vi "Load Default Configuration.vi"(8 "error in (no error)":errorcluster, 11 "CIFTemplatePlugin in":refnum<class "CIFTemplatePlugin.lvclass">) -> (0 "error out":errorcluster, 3 "CIFTemplatePlugin out":refnum<class "CIFTemplatePlugin.lvclass">)   [LabVIEW 2021, in "CIFTemplatePlugin.lvclass"]
uses:
  CIFTemplatePlugin.lvclass
  D:/dev/CIF-LVCore/src/CIFCore/Class/CIFCorePlugin.lvclass
  CIFCore/Common/Typedef/Common Plugin Configuration.ctl
  CIFTemplatePlugin.lvclass/CIFTemplatePlugin.ctl
  CIFCore/Class/CIFCorePlugin.lvclass/CIFCorePlugin.ctl
  CIFUtilities/CIFOutOfBand/CIFOutOfBand.lvclass/CIFOutOfBand.ctl
  CIFUtilities/CIFClocks/Core/Get Time.vi
  <vilib>/Utility/error.llb/Clear Errors.vi
  CIFCore/OOB/OOB_Rx/Load Payload.vi
  CIFCore/Class/Accessors/Read Plugin Name.vi
  CIFUtilities/CIFClocks/Time Conversion/LabVIEW Time to UTC Time.vi
  CIFUtilities/CIFClocks/SubVIs/Add Error.vi
  CIFUtilities/CIFOutOfBand/Accessors/Write Local OOB Data.vi
  CIFUtilities/CIFOutOfBand/Accessors/Read Local OOB Data.vi
  CIFCore/Common/Utilities/Append Error Location.vi
  CIFCore/OOB/OOB_Rx/CIFCoreOOB_Rx.lvclass
  D:/dev/CIF-LVCore/src/CIFUtilities/CIFOutOfBand/CIFOutOfBand.lvclass
  <vilib>/addons/_JKI.lib/Serialization/JSON/Library/Flatten To JSON String.vi
  CIFUtilities/CIFLogs/Logs/Write JSON to Config.vi
  CIFCore/Common/CIFCoreCommon.lvlib
  CIFCore/Class/CIFCorePlugin.lvclass
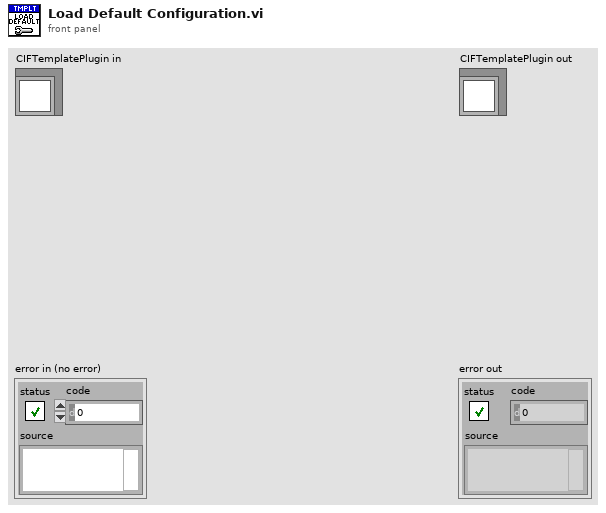
[diagram p1: front panel]
types:
  T1 = typedef "CIFCoreCommon.lvlib/Common Plugin Configuration.ctl" = cluster{"Period (s)":dbl, "Offset (us)":i32, "ClockID":u8, "Priority":i32, "Processor":i32}
  T2 = typedef "CIFTemplatePluginCommon.lvlib/Configuration.ctl" = cluster{"Common":T1, "Step":u64}
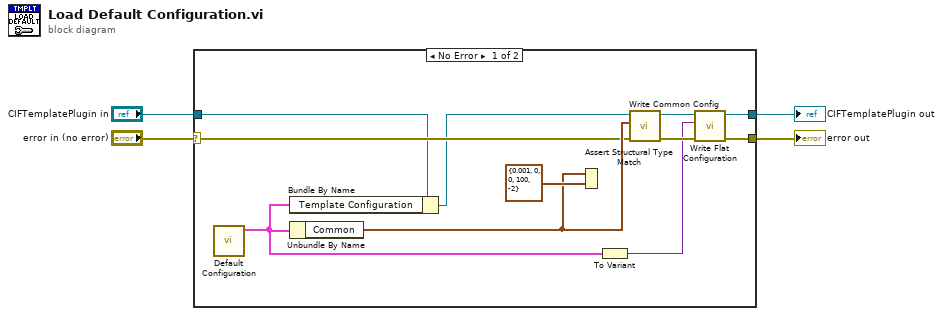
[diagram p0: block diagram]
diagram:
  n1 = case shown="No Error" "error in (no error)" {
    selector: "error in (no error)" -> [w8 w16]
    tunnel: "CIFTemplatePlugin in" -> [w7 w17]
    tunnel: [w11 w17] -> w1
    tunnel: [w10 w16] -> w3
    frame No Error {
      n2 = call "Default Configuration.vi"() -> ("Default Configuration"=w6:T2)  [unwired: 11 in]
      n3 = Bundle By Name(cluster=w7, "Template Configuration"=w6) -> (w5:refnum<class "CIFTemplatePlugin.lvclass">)
      n4 = Unbundle By Name(w6) -> ("Common"=w14:T1)
      n5 = Assert Structural Type Match(0:T1 {"Period (s)"=0.001, "Offset (us)"=0, "ClockID"=0, "Priority"=100, "Processor"=-2} ("Common"), 1:w14) -> ()
      n6 = To Variant(anything=w6) -> (Variant=w9:variant)
      n7 = call "Write Common Config.vi"("error in (no error)"=w8, "Common"=w14, "CIFTemplateNode in"=w5) -> ("error out"=w12:errorcluster, "CIFTemplateNode out"=w13:refnum<class "CIFTemplatePlugin.lvclass">)  [unwired: 7 in]
      n8 = call "Write Flat Configuration.vi"("error in (no error)"=w12, "Configuration"=w9, "CIFTemplateNode in"=w13) -> ("error out"=w10:errorcluster, "CIFTemplateNode out"=w11:refnum<class "CIFTemplatePlugin.lvclass">)  [unwired: 7 in]
    }
    frame Error {
    }
  }
  "error out" <- w3
  "CIFTemplatePlugin out" <- w1
